vi "Queue Init.vi"(9 "Queue Self":map{string, refnum<data-value>}(c390), 10 "Queue Caller":map{string, refnum<data-value>}(c390)) -> (3 "jettl Queue Actor out":refnum<class "jettl Queue Actor.lvclass">)   [LabVIEW 2021, in "jettl.lvlib" / "jettl Queue Actor.lvclass"]
uses:
  jettl Queue Actor.lvclass
  Actor/Msg/Msg.lvclass
  Queue State/Nominal Queue State/Nominal Queue State.lvclass
  C:/git/jettl/src/jettl/Queue State/Queue State/Queue State.lvclass
  jettl Queue Actor.lvclass/jettl Queue Actor.ctl
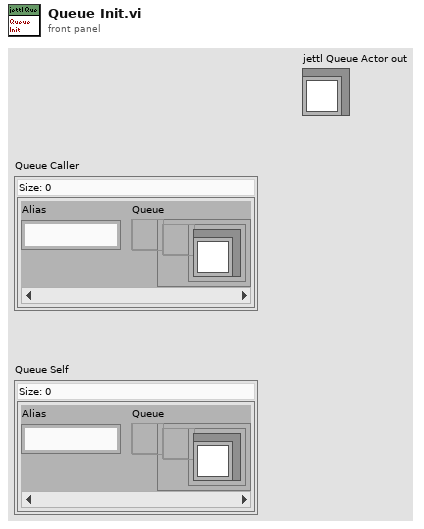
[diagram p1: front panel]
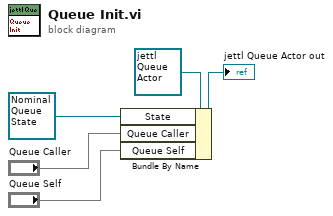
[diagram p0: block diagram]
diagram:
  n1 = Bundle By Name(cluster=refnum<class "jettl Queue Actor.lvclass"> refnum ("Self Actor in"), "State"=refnum<class "Nominal Queue State.lvclass"> refnum ("LVCAM.lvlib:Msging Self Actor State.lvclass"), "Queue Caller"="Queue Caller", "Queue Self"="Queue Self") -> (→"jettl Queue Actor out":refnum<class "jettl Queue Actor.lvclass">)
